vi "Error_MergeErrors.vi"(0 "error in 1":errorcluster, 1 "error in 2":errorcluster, 2 "errorArray":errorcluster[](array[cluster])) -> (15 "allErrorOut":errorcluster[](array[cluster]), 19 "error out":errorcluster)   [LabVIEW 2017]
doc: "Searches for errors in the incoming errorclusters. First error1 then error2, last errorarray."
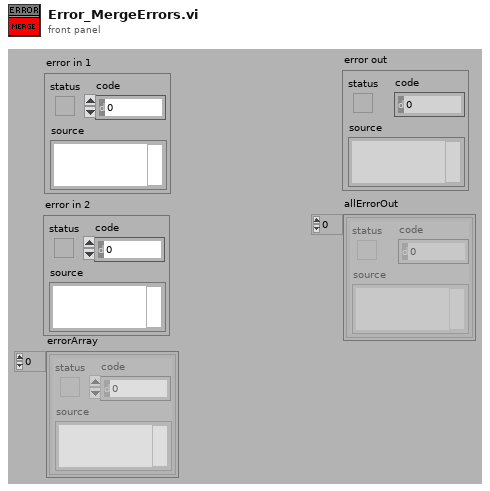
[diagram p1: front panel]
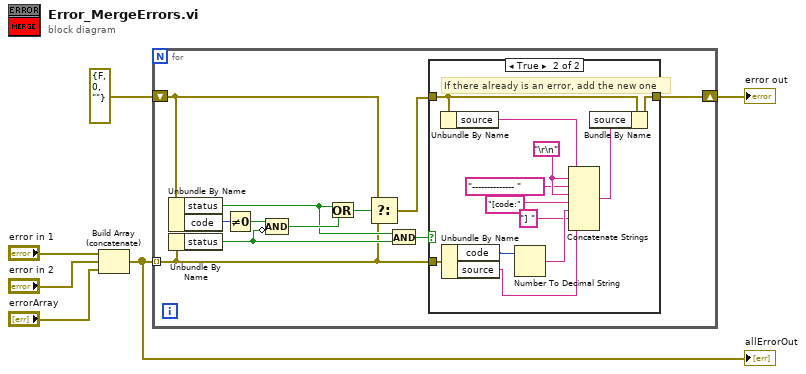
[diagram p0: block diagram]
diagram:
  n1 = Build Array (concatenate)("error in 1", "error in 2", "errorArray") -> (w1:errorcluster[])
  "allErrorOut" <- w1
  n2 = for {
    tunnel: w1 -> [w7] mode=indexing
    shift-right: [w11] -> w2
    shift-left: errorcluster {"status"=FALSE, "code"=0, "source"=""} ("error in (no error)") -> [w17]
    n3 = Unbundle By Name(w17) -> ("status"=w9:bool, "code"=w15:i32)
    n4 = Unbundle By Name(w7) -> ("status"=w10:bool)
    n5 = Not Equal To 0?(x=w15) -> (x != 0?=w14:bool)
    n6 = Compound Arithmetic op=AND(w14, invert w10) -> (w13:bool)
    n7 = Or(x=w9, y=w13) -> (x .or. y?=w16:bool)
    n8 = Select(t=w17, s=w16, f=w7) -> (s? t:f=w12:errorcluster)
    n9 = And(x=w9, y=w10) -> (x .and. y?=w8:bool)
    n10 = case shown="True" w8 {
      tunnel: w12 -> [w18 w29]
      tunnel: [w18 w30] -> w11
      tunnel: w7 -> [_ w28]
      frame False {
      }
      frame True {
        w20 = "\r\n"
        # "If there already is an error, add the new one"
        n11 = Unbundle By Name(w29) -> ("source"=w21:string)
        n12 = Unbundle By Name(w28) -> ("code"=w26:i32, "source"=w22:string)
        n13 = Number To Decimal String(number=w26) -> (decimal integer string=w24:string)  [unwired: 1 out]
        n14 = Concatenate Strings(w21, w20, "-------------- ", w20, "[code:" ("Substring"), w24, "] " ("Substring"), w22) -> (w27:string)
        n15 = Bundle By Name(cluster=w29, "source"=w27) -> (w30:errorcluster)
      }
    }
  }
  "error out" <- w2
